vi "ConfigTrigger.vi"(8 "error in (no error)":errorcluster, 11 "ClassIn":refnum<class "Keysight335XX.lvclass">) -> (0 "error out":errorcluster, 3 "ClassOut":refnum<class "Keysight335XX.lvclass">)   [LabVIEW 2014, in "FGenPlugins.lvlib" / "Keysight335XX.lvclass"]
uses:
  Keysight335XX.lvclass
  MyPluginBaseClass/TypeDef/ChannelParamElement.ctl
  <instrlib>/Agilent 3352X Series/Agilent 3352X Series.lvlib
  MyPluginBaseClass/NISTFGenPluginsBase.lvclass
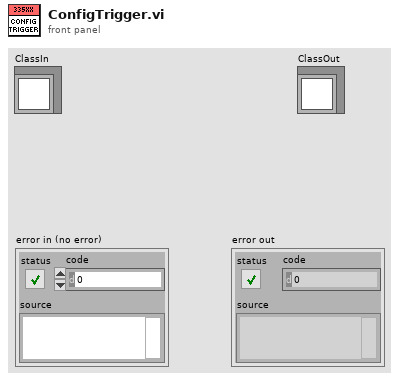
[diagram p1: front panel]
types:
  T1 = typedef "NISTFGenPlugins.lvlib/NISTFGenPluginsBase.lvclass/TriggerParams.ctl" = cluster{"eTrigger":u16, "eEdge":u16, "sSource":string}
  T2 = typedef "FGenPlugins.lvlib/NISTFGenPluginsBase.lvclass/ChannelParamElement.ctl" = cluster{"sName":string, "eOperateMode":u16, "bEnabled":bool, "eOutputMode":u16, "iIndex":i32, "iNameBufferSize":i32, "fGain":dbl}
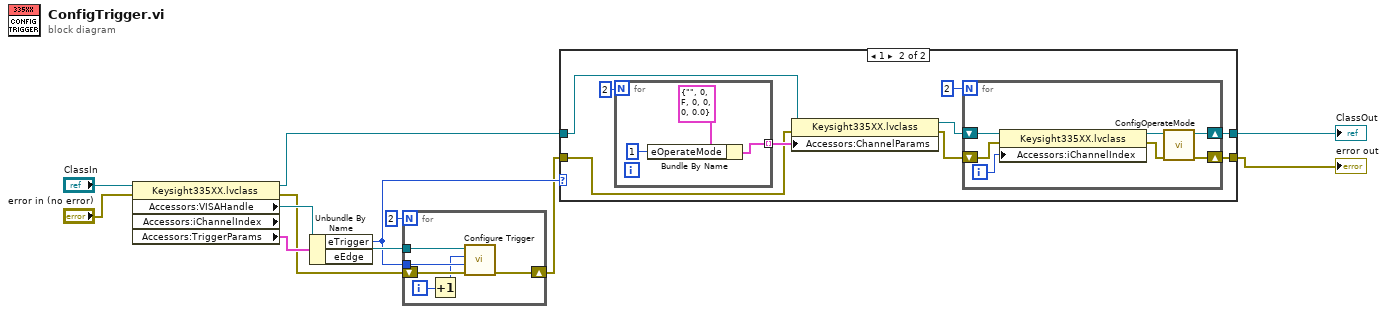
[diagram p0: block diagram]
diagram:
  n1 = property class="Keysight335XX.lvclass" props=["Accessors:VISAHandle", "Accessors:iChannelIndex", "Accessors:TriggerParams"](reference="ClassIn", error in="error in (no error)") -> (reference out=w7:refnum<class "Keysight335XX.lvclass">, error out=w2:errorcluster, "Accessors:VISAHandle"=w9:refnum<visa-resource-name>, "Accessors:TriggerParams"=w8:T1)  [unwired: 1 out]
  n2 = Unbundle By Name(w8) -> ("eTrigger"=w4:u16)  [unwired: 1 out]
  n3 = for {
    N: 2 -> [_]
    tunnel: w9 -> [w17]
    tunnel: w4 -> [w15]
    shift-right: [w16] -> w1
    shift-left: w2 -> [w14]
    i -> [w13]
    n4 = Increment(x=w13) -> (x+1=w12:i32)
    n5 = call <instrlib>:"Configure Trigger.vi"("error in (no error)"=w14, "Trigger Source (0: Immediate)"=w15, "Channel (1: 1)"=w12, "VISA resource name"=w17) -> ("error out"=w16:errorcluster)  [unwired: 6 in, 1 out]
  }
  n6 = case shown="1" w4 {
    tunnel: w7 -> [w19 w25]
    tunnel: w1 -> [w18 w23]
    tunnel: [w18 w28] -> w3
    tunnel: [w19 w27] -> w6
    frame 0, Default {
    }
    frame 1 {
      n7 = for {
        N: 2 -> [_]
        tunnel: [w36] -> w24 mode=indexing
        n8 = Bundle By Name(cluster=T2 {"sName"="", "eOperateMode"=0, "bEnabled"=FALSE, "eOutputMode"=0, "iIndex"=0, "iNameBufferSize"=0, "fGain"=0.0} ("ChannelParamElement"), "eOperateMode"=u16 1) -> (w36:T2)
      }
      n9 = property class="Keysight335XX.lvclass"(reference=w25, error in=w23, "Accessors:ChannelParams"=w24) -> (reference out=w22:refnum<class "Keysight335XX.lvclass">, error out=w21:errorcluster)
      n10 = for {
        N: 2 -> [_]
        shift-right: [w34] -> w27
        shift-left: w22 -> [w33]
        shift-right: [w35] -> w28
        shift-left: w21 -> [w32]
        i -> [w29]
        n11 = property class="Keysight335XX.lvclass"(reference=w33, error in=w32, "Accessors:iChannelIndex"=w29) -> (reference out=w31:refnum<class "Keysight335XX.lvclass">, error out=w30:errorcluster)
        n12 = call-dynamic "ConfigOperateMode.vi"("error in (no error)"=w30, "ClassIn"=w31) -> ("error out"=w35:errorcluster, "ClassOut"=w34:refnum<class "Keysight335XX.lvclass">)  [unwired: 8 in]
      }
    }
  }
  "error out" <- w3
  "ClassOut" <- w6
